vi "ConnectionDataRead.vi"(8 "error in (no error)":errorcluster, 9 "ReadData":refnum<class "ReadData.lvclass">, 10 "Connection":refnum<class "Connection.lvclass">, 11 "Tcp in":refnum<class "Tcp.lvclass">) -> (0 "error out":errorcluster, 3 "Tcp out":refnum<class "Tcp.lvclass">)   [LabVIEW 2022 SP3, in "Tcp.lvlib" / "Tcp.lvclass"]
uses:
  Tcp.lvclass
  DataReceived/DataReceived.lvclass
  CallerMessage Messages/TcpDataReceived Msg/TcpDataReceived Msg.lvclass
  <vilib>/ActorFramework/Actor/Actor.lvclass
  Connection/ReadData/ReadData.lvclass
  TcpSocket/Source/TcpSocket/Connection/Connection.lvclass
  C:/Program Files (x86)/National Instruments/LabVIEW 2022/vi.lib/ActorFramework/Actor/Actor.lvclass
  C:/Users/jakub/repos/gh/lv-cli-example/Source/Tcp/Tcp/Tcp.lvclass
  C:/Users/jakub/repos/gh/lv-cli-example/Source/Connection/CallerMessage/CallerMessage.lvclass
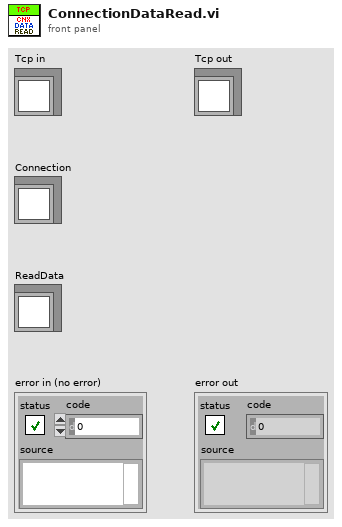
[diagram p1: front panel]
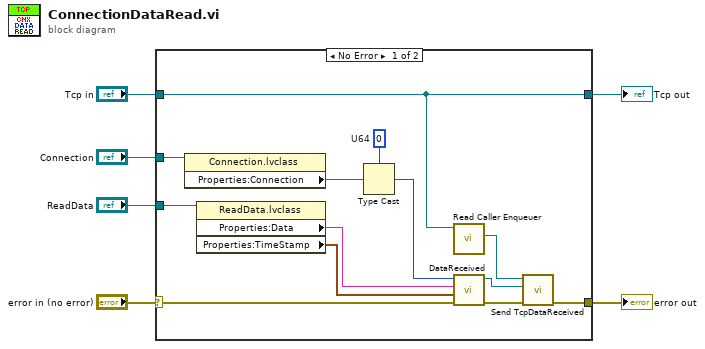
[diagram p0: block diagram]
diagram:
  n1 = case shown="No Error" "error in (no error)" {
    selector: "error in (no error)" -> [w8 w21]
    tunnel: "ReadData" -> [w19 _]
    tunnel: "Connection" -> [w18 _]
    tunnel: [w11 w21] -> w4
    tunnel: "Tcp in" -> [w7 w20]
    tunnel: [w7 w20] -> w1
    frame No Error {
      w16 = u64 0  # U64
      n2 = property class="Connection.lvclass"(reference=w18) -> ("Properties:Connection"=w17:refnum<k5>)  [unwired: 1 in, 2 out]
      n3 = property class="ReadData.lvclass"(reference=w19) -> ("Properties:Data"=w14:string, "Properties:TimeStamp"=w13:timestamp)  [unwired: 1 in, 2 out]
      n4 = Type Cast(type=w16, x=w17) -> (*(type *) &x=w15:u64)
      n5 = call <vilib>:"Read Caller Enqueuer.vi"("Actor"=w7) -> ("Caller Enqueuer"=w10:refnum<class "Message Enqueuer.lvclass">)  [unwired: 10 in]
      n6 = call "DataReceived.vi"("error in (no error)"=w8, "TimeStamp"=w13, "Data"=w14, "Refnum"=w15) -> ("error out"=w12:errorcluster, "DataReceived"=w9:refnum<class "DataReceived.lvclass">)  [unwired: 6 in]
      n7 = call "Send TcpDataReceived.vi"("error in (no error)"=w12, "DataReceived"=w9, "Message Enqueuer"=w10) -> ("error out"=w11:errorcluster)  [unwired: 7 in, 1 out]
    }
    frame Error {
    }
  }
  "error out" <- w4
  "Tcp out" <- w1
